vi "inverse s-box.vi"(0 "x":dbl[](array[numeric]), 1 "y":dbl[](array[numeric]), 2 "z":dbl[](array[numeric]), 3 "red in":dbl[](array[numeric]), 4 "green in":dbl[](array[numeric]), 5 "blue in":dbl[](array[numeric]), 6 "Numeric":i32) -> (15 "red out":u8[](array[numeric]), 16 "green out":u8[](array[numeric]), 17 "blue out":u8[](array[numeric]))   [LabVIEW 2019]
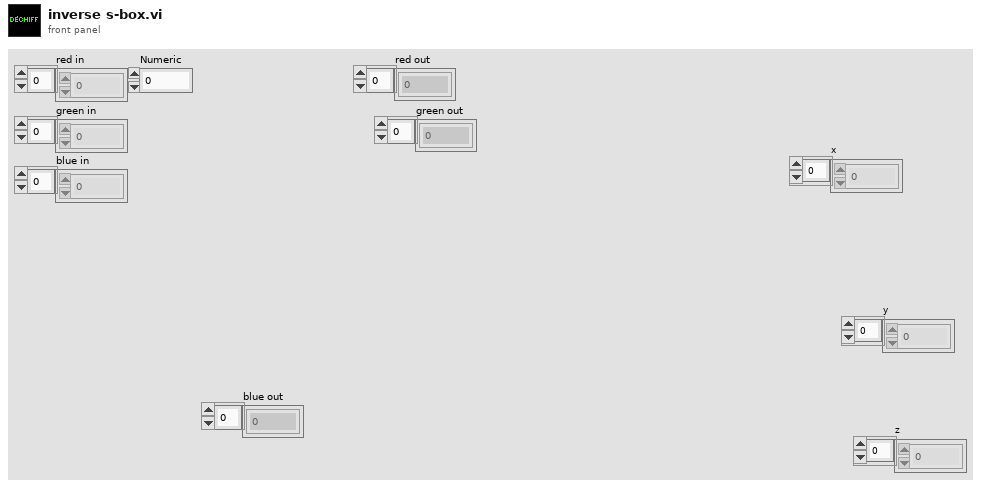
[diagram p1: front panel]
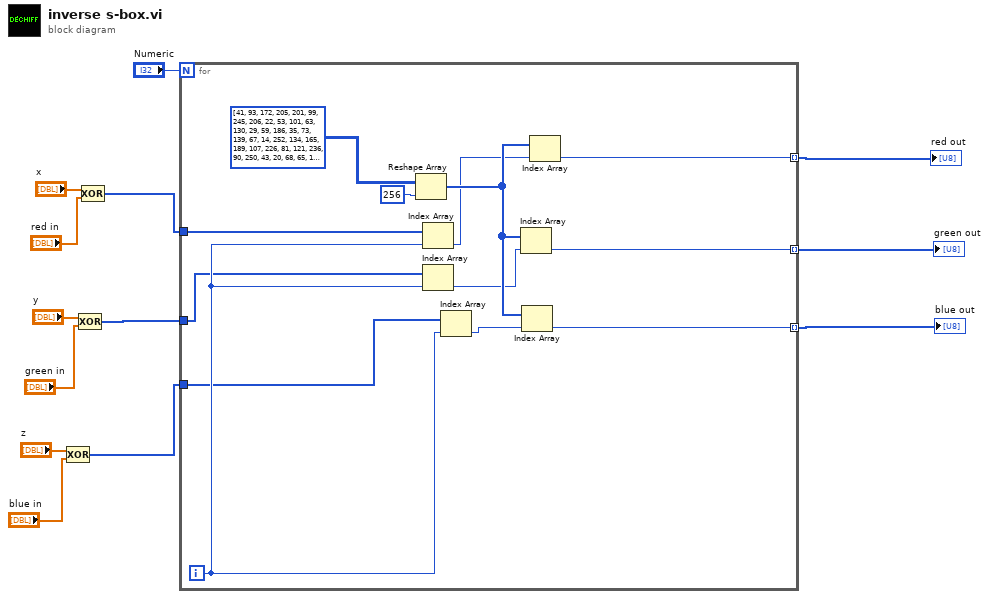
[diagram p0: block diagram]
diagram:
  n1 = Compound Arithmetic op=XOR("z", "blue in") -> (w4:i32[])
  n2 = Compound Arithmetic op=XOR("y", "green in") -> (w6:i32[])
  n3 = Compound Arithmetic op=XOR("x", "red in") -> (w8:i32[])
  n4 = for {
    N: "Numeric" -> [_]
    tunnel: [w19] -> w12 mode=indexing
    tunnel: [w18] -> w13 mode=indexing
    tunnel: [w17] -> w11 mode=indexing
    tunnel: w8 -> [w16]
    tunnel: w6 -> [w15]
    tunnel: w4 -> [w14]
    i -> [w20]
    n5 = Reshape Array(u8[][] [[41, 93, 172, 205, 201, 99, 245, 206, 22, 53, 101, 63, 130, 29, 59, 186], [35, 73, 139, 67, 14, 252, 134, 165, 189, 107, 226, 81, 121, 236, 90, 250], [43, 20, 68, 65, 103, 23, 251, 191, 62, 207, 17, 155, 52, 237, 8, 96], [7, 19, 243, 47, 1, 169, 79, 177, 119, 5, 91, 235, 246, 176, 168, 0], [117, 88, 129, 214, 45, 26, 111, 181, 145, 30, 249, 32, 71, 144, 69, 124], [166, 188, 153, 18, 31, 104, 70, 221, 28, 149, 202, 217, 194, 254, 212, 74], [42, 25, 44, 158, 179, 239, 247, 95, 114, 9, 137, 203, 100, 190, 192, 229], [83, 13, 126, 56, 174, 10, 162, 142, 48, 112, 222, 66, 127, 89, 132, 2], [195, 198, 147, 223, 232, 187, 85, 161, 36, 21, 51, 40, 228, 220, 156, 76], [159, 120, 15, 61, 241, 105, 154, 173, 244, 75, 255, 77, 50, 219, 33, 175], [233, 57, 109, 46, 218, 160, 118, 64, 148, 12, 138, 123, 152, 151, 122, 242], [39, 113, 78, 178, 110, 196, 141, 135, 72, 150, 11, 116, 185, 125, 143, 55], [216, 60, 146, 248, 115, 209, 183, 92, 87, 230, 184, 98, 167, 131, 163, 215], [24, 200, 136, 225, 193, 4, 38, 210, 84, 34, 208, 234, 164, 58, 106, 227], [16, 171, 240, 80, 49, 170, 82, 157, 102, 197, 128, 54, 6, 211, 97, 199], [238, 231, 224, 37, 94, 133, 180, 27, 86, 3, 140, 204, 253, 182, 213, 108]], 256 ("dimension size")) -> (w26:u8[])
    n6 = Index Array(array=w16, index=w20) -> (element=w23:i32)
    n7 = Index Array(array=w15, index=w20) -> (element=w22:i32)
    n8 = Index Array(array=w14, index=w20) -> (element=w21:i32)
    n9 = Index Array(array=w26, index=w22) -> (element=w19:u8)
    n10 = Index Array(array=w26, index=w21) -> (element=w17:u8)
    n11 = Index Array(array=w26, index=w23) -> (element=w18:u8)
  }
  "red out" <- w13
  "green out" <- w12
  "blue out" <- w11
